vi "Integer Field To String.vi"(8 "error in (no error)":errorcluster, 11 "Sudoku Class in":refnum<class "Sudoku Class.lvclass">) -> (0 "error out":errorcluster, 2 "Sudoku String":T1, 3 "Sudoku Class out":refnum<class "Sudoku Class.lvclass">)   [LabVIEW 2015, in "Sudoku Library.lvlib" / "Sudoku Class.lvclass"]
doc: "Created IvanLis by LabVIEW Portal\nProfile: http://labviewportal.org/memberlist.php?mode=viewprofile&u=987\neMail: IvanLisanov@gMail.com\nTelegram: https://t.me/IvanLis"
uses:
  Sudoku Class.lvclass
  TypeDef/Sudoku String.ctl
  Sudoku Class.lvclass/Sudoku Class.ctl
  Sudoku Library.lvlib
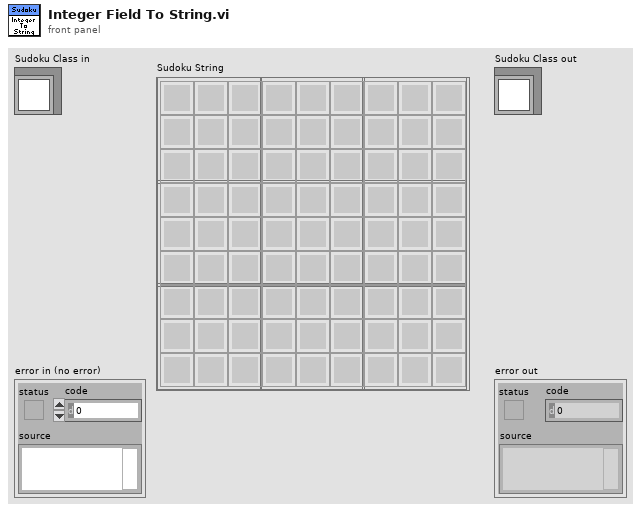
[diagram p1: front panel]
types:
  T1 = typedef "Sudoku Library.lvlib/Sudoku String.ctl" = string[][]
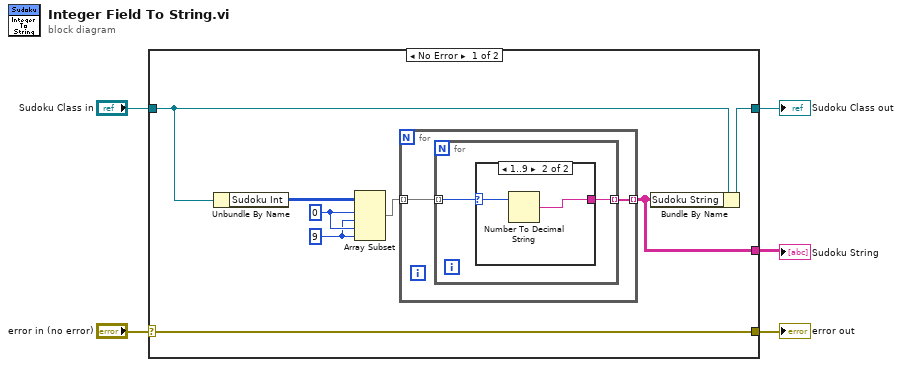
[diagram p0: block diagram]
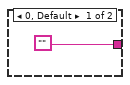
[diagram p2: hidden frame]
diagram:
  n1 = case shown="No Error" "error in (no error)" {
    selector: "error in (no error)" -> [w10 w22]
    tunnel: [w10 w22] -> w4
    tunnel: [w11 w21] -> w2
    tunnel: "Sudoku Class in" -> [w13 w21]
    tunnel: [w9 _] -> w1
    frame No Error {
      w6 = 9 ("length")
      w7 = 0 ("index")
      n2 = Unbundle By Name(w13) -> ("Sudoku Int"=w12:u8[][])
      n3 = Array Subset(array=w12, index (row)=w7, length (row)=w6, index (col)=w7, length (col)=w6) -> (w8:u8[][])
      n4 = for {
        tunnel: w8 -> [w15] mode=indexing
        tunnel: [w14] -> w9 mode=indexing
        n5 = for {
          tunnel: w15 -> [w16] mode=indexing
          tunnel: [w17] -> w14 mode=indexing
          n6 = case shown="1..9" w16 {
            selector: w16 -> [_ w20]
            tunnel: ["" w19] -> w17
            frame 0, Default {
            }
            frame 1..9 {
              n7 = Number To Decimal String(number=w20) -> (decimal integer string=w19:string)  [unwired: 1 in]
            }
          }
        }
      }
      n8 = Bundle By Name(cluster=w13, "Sudoku String"=w9) -> (w11:refnum<class "Sudoku Class.lvclass">)
    }
    frame Error {
    }
  }
  "error out" <- w4
  "Sudoku Class out" <- w2
  "Sudoku String" <- w1
